vi "MAIN_merFISH_wait_for_stabilization.vi"(5 "queue ASI stage":refnum<queue>, 6 "error in":errorcluster, 7 "Measure QPD":bool caption="Calibration", 8 "Data cluster":T1, 9 "queue piezo":refnum<queue>) -> (0 "error out":errorcluster, 3 "Next task":T2)   [LabVIEW 2015]
uses:
  CONTROLS/Q_main_element.ctl
  CONTROLS/Q_MCL_piezo_element.ctl
  CONTROLS/Q_ASI_stage_element.ctl
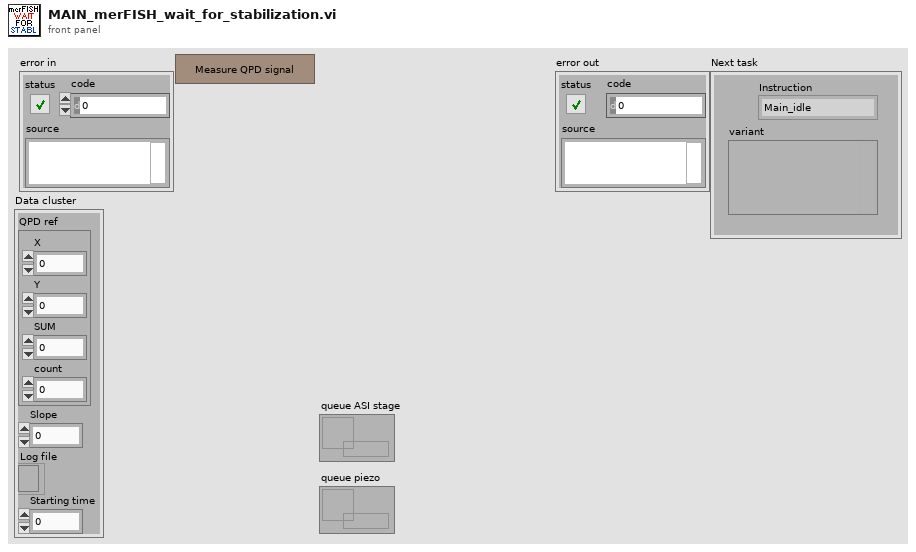
[diagram p1: front panel]
types:
  T1 = cluster{"QPD ref":cluster{"X":sgl, "Y":sgl, "SUM":sgl, "count":u32}, "Slope":dbl, "Log file":refnum<file>, "Starting time":dbl}
  T2 = typedef "Q_main_element.ctl" = cluster{"variant":variant, "Instruction":enum16{"Main_idle", "Main_initialize", "Main_initialize_TDMS", "Main_initialize_Queue", "Main_error", "Main_DAQ_initialization_results", "Main_ASI_initialization_results", "Main_Piezo_initialization_results", "Main_Valve_initialization_results", "Main_Pump_initialization_results", "Main_CAMERA_initialization_results", "Main_FPGA_initialization_results", "Main_DAQ_error", "Main_ASI_error", "Main_Piezo_error", "Main_CAMERA_error", "Main_Valve_error", "Main_Pump_error", "Main_FPGA_error", "Main_start_acquiring", "Main_not_acquiring", "Main_acquiring", "Main_stop_acquiring", "Main_change_exposure", "Main_change_z_scan_parameters", "Main_define_ROI", "Main_define_mosaic", "Main_read_kinetic_time", "Main_cooler", "Main_read_temperature", "Main_save_XY", "Main_load_XY", "Main_discard_XY", "Main_move_to_XY", "Main_measure_QPD", "Main_autofocus_calibration", "Main_autofocus_initialization", "Main_autofocus_stop", "Main_save_PID", "Main_change_H_valve_position", "Main_two_way_valve", "Main_save_movie", "Main_init_single_scan", "Main_single_scan", "Main_stop_single_scan", "Main_merFISH_illumination_parameters", "Main_merFISH_buffer_probe_list", "Main_merFISH_injections_procedure", "Main_merFISH_save_setpoint", "Main_merFISH_DAPI_parameters", "Main_merFISH_Brightfield_parameters", "Main_merFISH_save_embryo_ROI", "Main_merFISH_init", "Main_merFISH_resume", "Main_merFISH_start_autofocus", "Main_merFISH_open_close_valve_merFISH", "Main_merFISH_open_close_valve_photobleaching", "Main_merFISH_hybridization", "Main_merFISH_move_to_ROI", "Main_merFISH_wait_stabilization", "Main_merFISH_move_to_REF", "Main_merFISH_scan", "Main_merFISH_photobleaching_injection", "Main_merFISH_photobleaching", "Main_merFISH_send_email", "Main_merFISH_close", "Main_STOP"}}
  T3 = cluster{"QPD ref":cluster{"X":sgl, "Y":sgl, "SUM":sgl, "count":u32}, "Slope":dbl}
  T4 = cluster{"X":sgl, "Y":sgl, "SUM":sgl, "count":u32}
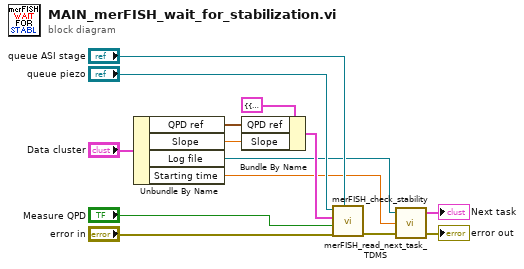
[diagram p0: block diagram]
diagram:
  n1 = Unbundle By Name("Data cluster") -> ("QPD ref"=w5:T4, "Slope"=w4:dbl, "Log file"=w3:refnum<file>, "Starting time"=w2:dbl)
  n2 = Bundle By Name(cluster=T3 {"QPD ref"={"X"=0.0, "Y"=0.0, "SUM"=0.0, "count"=0}, "Slope"=0.0} ("Data cluster"), "QPD ref"=w5, "Slope"=w4) -> (w13:T3)
  n3 = call "merFISH_check_stability.vi"("queue ASI stage"="queue ASI stage", "error in"="error in", "Measure QPD"="Measure QPD", "Data cluster"=w13, "queue piezo"="queue piezo") -> ("error out"=w14:errorcluster)  [unwired: 4 in]
  n4 = call "merFISH_read_next_task_TDMS.vi"("error in"=w14, "Starting time"=w2, "Log file"=w3) -> ("error out"=→"error out":errorcluster, "task"=→"Next task":T2)  [unwired: 1 in]
